vi "SetLocalPoseDecode.vi"(0 "Payload":string) -> (2 "PresenceVector":u16=2 format="%b", 3 "LocalPose":T1)   [LabVIEW 2009]
uses:
  Support Files/LocalPose.ctl
  Support Files/TimeRec.ctl
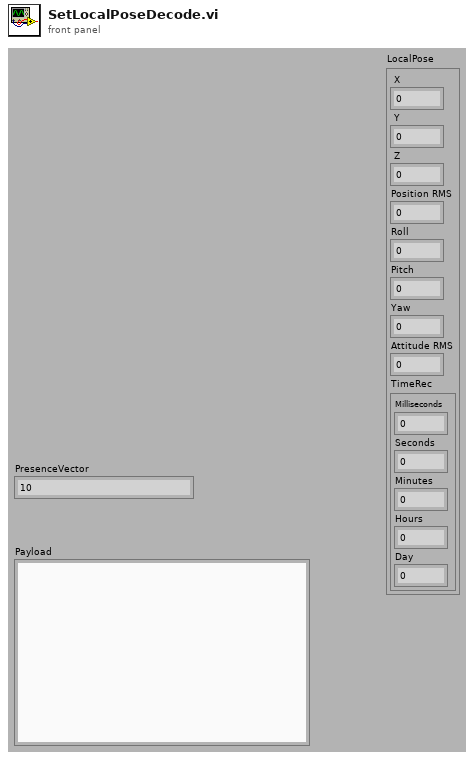
[diagram p1: front panel]
types:
  T1 = typedef "LocalPose.ctl" = cluster{" X":dbl, " Y":dbl, " Z":dbl, "Position RMS":dbl, "Roll":dbl, "Pitch":dbl, "Yaw":dbl, "Attitude RMS":dbl, "TimeRec":T2}
  T2 = typedef "TimeRec.ctl" = cluster{"Milliseconds":u32, "Seconds":u32, "Minutes":u32, "Hours":u32, "Day":u32}
  T3 = cluster{"unsigned byte array[0]":u8, "unsigned byte array[1]":u8}
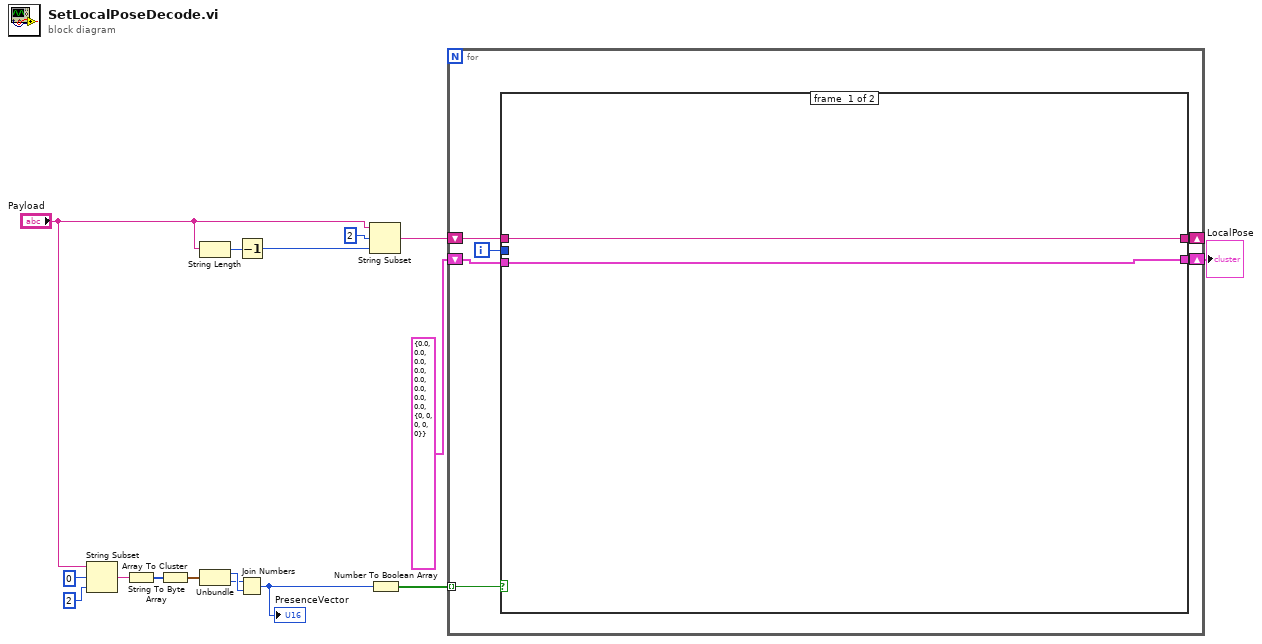
[diagram p0: block diagram]
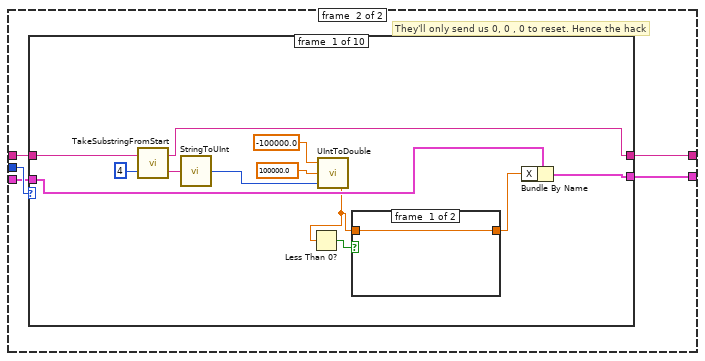
[diagram p2: hidden frame]
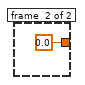
[diagram p3: hidden frame]
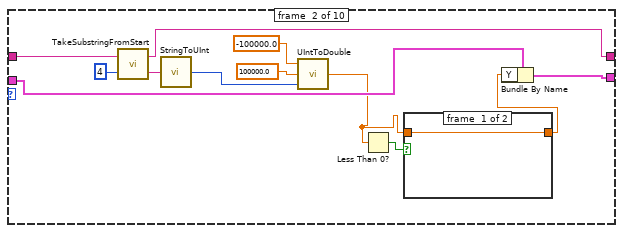
[diagram p4: hidden frame]
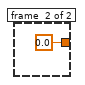
[diagram p5: hidden frame]
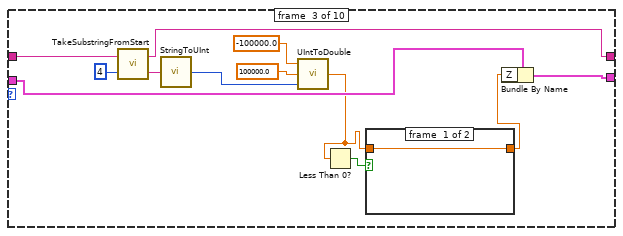
[diagram p6: hidden frame]
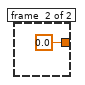
[diagram p7: hidden frame]
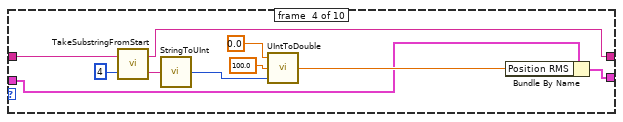
[diagram p8: hidden frame]
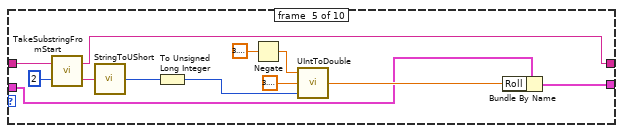
[diagram p9: hidden frame]
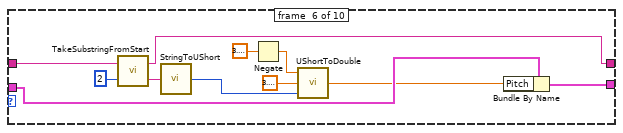
[diagram p10: hidden frame]
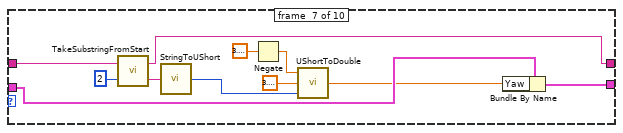
[diagram p11: hidden frame]
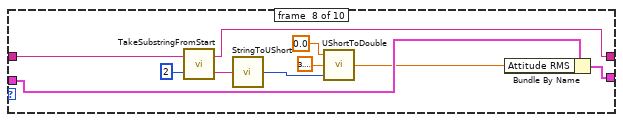
[diagram p12: hidden frame]
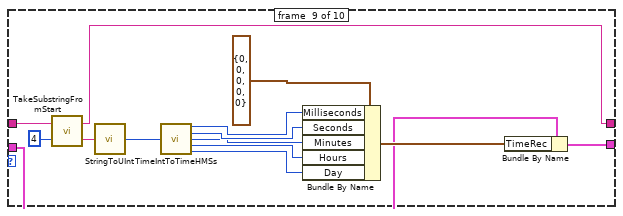
[diagram p13: hidden frame]
diagram:
  n1 = String Subset(string="Payload", offset (0)=0, length (rest)=2 ("length (rest)")) -> (substring=w11:string)
  n2 = String To Byte Array(string=w11) -> (unsigned byte array=w10:u8[])
  n3 = Array To Cluster(array=w10) -> (cluster=w9:T3)
  n4 = String Length(string="Payload") -> (length=w4:i32)
  n5 = Unbundle(w9) -> ("unsigned byte array[0]"=w8:u8, "unsigned byte array[1]"=w7:u8)
  n6 = Decrement(x=w4) -> (x-1=w5:i32)
  n7 = Join Numbers(hi=w7, lo=w8) -> ((hi.lo)=w6:u16)
  "PresenceVector" <- w6
  n8 = String Subset(string="Payload", offset (0)=2, length (rest)=w5) -> (substring=w15:string)
  n9 = Number To Boolean Array(number=w6) -> (Boolean array=w16:bool[])
  n10 = for {
    tunnel: w16 -> [w21] mode=indexing
    shift-right: [w19] -> _
    shift-left: w15 -> [w20]
    shift-right: [w17] -> w1
    shift-left: T1 {" X"=0.0, " Y"=0.0, " Z"=0.0, "Position RMS"=0.0, "Roll"=0.0, "Pitch"=0.0, "Yaw"=0.0, "Attitude RMS"=0.0, "TimeRec"={"Milliseconds"=0, "Seconds"=0, "Minutes"=0, "Hours"=0, "Day"=0}} ("LocalPose") -> [w18]
    i -> [w22]
    n11 = case shown="True" w21 {
      tunnel: w22 -> [_ w29]
      tunnel: w20 -> [w24 w28]
      tunnel: [w23 w27] -> w17
      tunnel: [w24 w26] -> w19
      tunnel: w18 -> [w23 w25]
      frame #0 {
      }
      frame #1 {
        # "They'll only send us 0, 0 , 0 to reset. Hence the hack"
        n12 = case shown="2" w29 {
          tunnel: w28 -> [w40 w54 w68 w80 w92 w103 w114 w124 w138 w141]
          tunnel: [w36 w48 w62 w72 w82 w101 w111 w123 w128 w140] -> w27
          tunnel: [w34 w50 w63 w76 w86 w98 w110 w116 w127 w141] -> w26
          tunnel: w25 -> [w33 w47 w61 w73 w83 w100 w112 w122 w129 w140]
          frame #0 {
            n13 = call "TakeSubstringFromStart.vi"("offset"=4 ("reduce by"), "string"=w40) -> ("string before offset"=w35:string, "string after offset"=w34:string)
            n14 = call "StringToUInt.vi"("string"=w35) -> ("UInt"=w39:u32)
            n15 = call "UIntToDouble.vi"("Value"=w39, "Max"=100000.0, "Min"=-100000.0) -> ("Number"=w31:dbl)
            n16 = Less Than 0?(x=w31) -> (x < 0?=w32:bool)
            n17 = case shown="True" w32 {
              tunnel: [w42 0.0 ("Number")] -> w30
              tunnel: w31 -> [w42 _]
              frame #0 {
              }
              frame #1 {
              }
            }
            n18 = Bundle By Name(cluster=w33, "X"=w30) -> (w36:T1)
          }
          frame #1 {
            n19 = call "TakeSubstringFromStart.vi"("offset"=4 ("reduce by"), "string"=w54) -> ("string before offset"=w49:string, "string after offset"=w50:string)
            n20 = call "StringToUInt.vi"("string"=w49) -> ("UInt"=w53:u32)
            n21 = call "UIntToDouble.vi"("Value"=w53, "Max"=100000.0, "Min"=-100000.0) -> ("Number"=w45:dbl)
            n22 = Less Than 0?(x=w45) -> (x < 0?=w46:bool)
            n23 = case shown="False" w46 {
              tunnel: [w56 0.0 ("Number")] -> w44
              tunnel: w45 -> [w56 _]
              frame #0 {
              }
              frame #1 {
              }
            }
            n24 = Bundle By Name(cluster=w47, "Y"=w44) -> (w48:T1)
          }
          frame #2 {
            n25 = call "TakeSubstringFromStart.vi"("offset"=4 ("reduce by"), "string"=w68) -> ("string before offset"=w64:string, "string after offset"=w63:string)
            n26 = call "StringToUInt.vi"("string"=w64) -> ("UInt"=w67:u32)
            n27 = call "UIntToDouble.vi"("Value"=w67, "Max"=100000.0, "Min"=-100000.0) -> ("Number"=w59:dbl)
            n28 = Less Than 0?(x=w59) -> (x < 0?=w60:bool)
            n29 = case shown="True" w60 {
              tunnel: [w70 0.0 ("Number")] -> w58
              tunnel: w59 -> [w70 _]
              frame #0 {
              }
              frame #1 {
              }
            }
            n30 = Bundle By Name(cluster=w61, "Z"=w58) -> (w62:T1)
          }
          frame #3 {
            n31 = call "TakeSubstringFromStart.vi"("offset"=4 ("reduce by"), "string"=w80) -> ("string before offset"=w75:string, "string after offset"=w76:string)
            n32 = call "StringToUInt.vi"("string"=w75) -> ("UInt"=w79:u32)
            n33 = call "UIntToDouble.vi"("Value"=w79, "Max"=100.0, "Min"=0.0) -> ("Number"=w74:dbl)
            n34 = Bundle By Name(cluster=w73, "Position RMS"=w74) -> (w72:T1)
          }
          frame #4 {
            n35 = call "TakeSubstringFromStart.vi"("offset"=2 ("reduce by"), "string"=w92) -> ("string before offset"=w85:string, "string after offset"=w86:string)
            n36 = call "StringToUShort.vi"("string"=w85) -> ("UShort"=w91:u16)
            n37 = To Unsigned Long Integer(number=w91) -> (unsigned 32bit integer=w87:u32)
            n38 = Negate(x=3.141592653589793) -> (-x=w89:dbl)
            n39 = call "UIntToDouble.vi"("Value"=w87, "Max"=3.141592653589793, "Min"=w89) -> ("Number"=w84:dbl)
            n40 = Bundle By Name(cluster=w83, "Roll"=w84) -> (w82:T1)
          }
          frame #5 {
            n41 = call "TakeSubstringFromStart.vi"("offset"=2 ("reduce by"), "string"=w103) -> ("string before offset"=w99:string, "string after offset"=w98:string)
            n42 = call "StringToUShort.vi"("string"=w99) -> ("UShort"=w95:u16)
            n43 = Negate(x=3.141592653589793) -> (-x=w97:dbl)
            n44 = call "UShortToDouble.vi"("Value"=w95, "Max"=3.141592653589793, "Min"=w97) -> ("Number"=w94:dbl)
            n45 = Bundle By Name(cluster=w100, "Pitch"=w94) -> (w101:T1)
          }
          frame #6 {
            n46 = call "TakeSubstringFromStart.vi"("offset"=2 ("reduce by"), "string"=w114) -> ("string before offset"=w109:string, "string after offset"=w110:string)
            n47 = call "StringToUShort.vi"("string"=w109) -> ("UShort"=w106:u16)
            n48 = Negate(x=3.141592653589793) -> (-x=w108:dbl)
            n49 = call "UShortToDouble.vi"("Value"=w106, "Max"=3.141592653589793, "Min"=w108) -> ("Number"=w105:dbl)
            n50 = Bundle By Name(cluster=w112, "Yaw"=w105) -> (w111:T1)
          }
          frame #7 {
            n51 = call "TakeSubstringFromStart.vi"("offset"=2 ("reduce by"), "string"=w124) -> ("string before offset"=w117:string, "string after offset"=w116:string)
            n52 = call "StringToUShort.vi"("string"=w117) -> ("UShort"=w119:u16)
            n53 = call "UShortToDouble.vi"("Value"=w119, "Max"=3.141592653589793, "Min"=0.0) -> ("Number"=w118:dbl)
            n54 = Bundle By Name(cluster=w122, "Attitude RMS"=w118) -> (w123:T1)
          }
          frame #8 {
            n55 = call "TakeSubstringFromStart.vi"("offset"=4 ("reduce by"), "string"=w138) -> ("string before offset"=w126:string, "string after offset"=w127:string)
            n56 = call "StringToUInt.vi"("string"=w126) -> ("UInt"=w137:u32)
            n57 = call "TimeIntToTimeHMSs.vi"("Time Int"=w137) -> ("Milliseconds"=w135:u32, "Seconds"=w134:u32, "Minutes"=w133:u32, "Hours"=w132:u32, "Day"=w131:u32)  [unwired: 10 in]
            n58 = Bundle By Name(cluster=T2 {"Milliseconds"=0, "Seconds"=0, "Minutes"=0, "Hours"=0, "Day"=0} ("TimeRec"), "Milliseconds"=w135, "Seconds"=w134, "Minutes"=w133, "Hours"=w132, "Day"=w131) -> (w130:T2)
            n59 = Bundle By Name(cluster=w129, "TimeRec"=w130) -> (w128:T1)
          }
          frame #9 {
          }
        }
      }
    }
  }
  "LocalPose" <- w1
